vi "Cache.Result.CheckNewData.vi"(8 "error in (no error)":errorcluster, 9 "max package size (25)":i32=25, 10 "Group in":string, 11 "tdms file in":refnum<k34>) -> (0 "error out":errorcluster, 1 "new data?":bool, 2 "Group out":string, 3 "tdms file out":refnum<k34>, 5 "offset":i64, 7 "records":bool[](array[boolean]))   [LabVIEW 2016]
panel:
  out "pos":i64
  out "channel length":i64
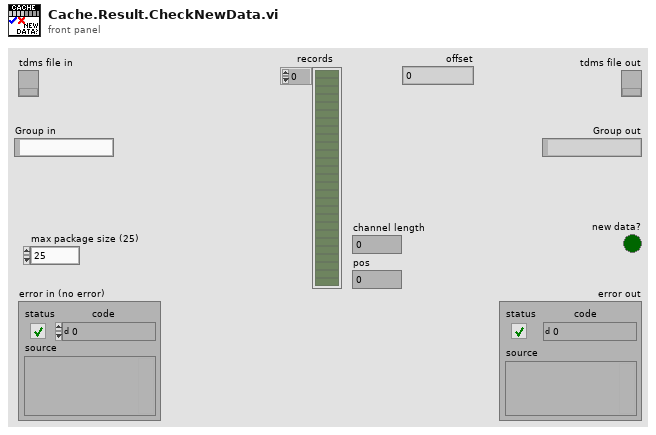
[diagram p1: front panel]
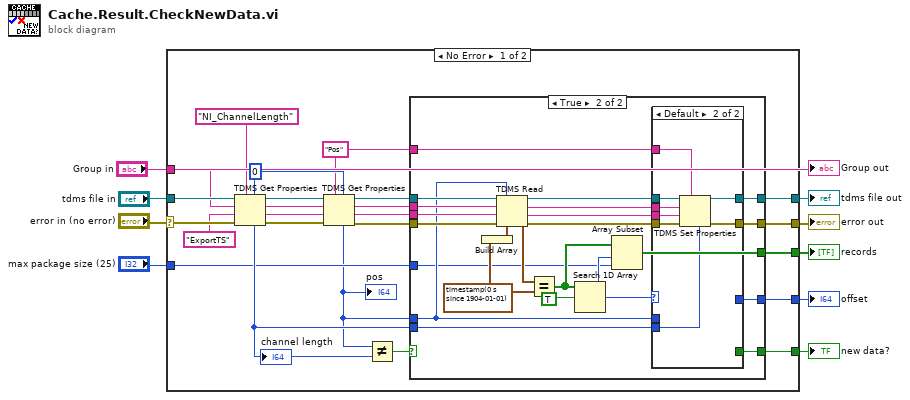
[diagram p0: block diagram]
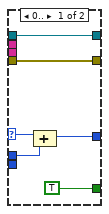
[diagram p3: hidden frame]
diagram:
  n1 = case shown="No Error" "error in (no error)" {
    selector: "error in (no error)" -> [w33 w74]
    tunnel: "tdms file in" -> [w32 w73]
    tunnel: [w18 w73] -> w8
    tunnel: [w17 w74] -> w7
    tunnel: "Group in" -> [w28 _]
    tunnel: [w14 _] -> w5
    tunnel: [w13 _] -> w4
    tunnel: [w12 _] -> w3
    tunnel: "max package size (25)" -> [w11 _]
    frame No Error {
      w27 = i64 0 ("pos")
      w15 = "Pos" ("channel name")
      n2 = TDMS Get Properties(5:w27, 7:"NI_ChannelLength" ("property name"), 8:w33, 9:"ExportTS" ("property names"), 10:w28, 11:w32) -> (0:w25:errorcluster, 1:w29:string, 2:w24:string, 3:w26:refnum<k34>, 4:w16:i64)  [unwired: 1 out]
      "channel length" <- w16
      n3 = TDMS Get Properties(5:w27, 7:w15, 8:w25, 9:w29, 10:w24, 11:w26) -> (0:w22:errorcluster, 1:w21:string, 2:w20:string, 3:w19:refnum<k34>, 4:w10:i64)  [unwired: 1 out]
      "pos" <- w10
      n4 = Not Equal?(x=w10, y=w16) -> (x != y?=w23:bool)
      n5 = case shown="True" w23 {
        tunnel: w22 -> [w34 w56]
        tunnel: w21 -> [_ w55]
        tunnel: w20 -> [_ w54]
        tunnel: w19 -> [w35 w53]
        tunnel: [w35 w47] -> w18
        tunnel: w10 -> [_ w49]
        tunnel: [w34 w50] -> w17
        tunnel: w16 -> [_ w46]
        tunnel: w15 -> [_ w45]
        tunnel: [_ w41] -> w14
        tunnel: [_ w40] -> w13
        tunnel: [_ w37] -> w12
        tunnel: w11 -> [_ w36]
        frame False {
        }
        frame True {
          w57 = timestamp(0 s since 1904-01-01) ("current time")
          n6 = Build Array(w57) -> (w58:timestamp[])
          n7 = TDMS Read(0:w53, 1:w49, 5:w54, 7:w55, 11:w56, 12:w58) -> (4:w48:refnum<k34>, 6:w44:string, 8:w42:string, 10:w43:timestamp[], 15:w51:errorcluster)  [unwired: 2 in, 1 out]
          n8 = Equal?(x=w43, y=w57) -> (x = y?=w39:bool[])
          n9 = Search 1D Array(1D array=w39, element=TRUE) -> (index of element=w38:i32)  [unwired: 1 in]
          n10 = Array Subset(array=w39, index=w38, length=w36) -> (w37:bool[])
          n11 = case shown="Default" w38 {
            selector: w38 -> [w63 _]
            tunnel: w51 -> [w64 w72]
            tunnel: [w64 w71] -> w50
            tunnel: w49 -> [w62 _]
            tunnel: w48 -> [w61 w70]
            tunnel: [w61 w69] -> w47
            tunnel: w46 -> [_ w68]
            tunnel: w45 -> [_ w67]
            tunnel: w44 -> [_ w66]
            tunnel: w42 -> [_ w65]
            tunnel: [w60 _] -> w41
            tunnel: [TRUE _] -> w40
            frame 0.. {
              n12 = Compound Arithmetic op=ADD(w63, w62) -> (w60:i64)
            }
            frame Default {
              n13 = TDMS Set Properties(5:w68, 7:w67, 8:w72, 9:w65, 10:w66, 11:w70) -> (0:w71:errorcluster, 3:w69:refnum<k34>)  [unwired: 2 out]
            }
          }
        }
      }
    }
    frame Error {
    }
  }
  "error out" <- w7
  "tdms file out" <- w8
  "offset" <- w5
  "new data?" <- w4
  "records" <- w3
  "Group out" <- "Group in"
